vi "S_ReadAttribute.vi"(8 "error in (no error)":errorcluster, 11 "reference in":refnum<class "SubTemplate_4x4x4.lvclass">) -> (0 "error out":errorcluster, 3 "reference out":refnum<class "SubTemplate_4x4x4.lvclass">)   [LabVIEW 2012, in "SubTemplate_4x4x4.lvclass"]
uses:
  <resource>/Framework/Providers/Open_GDS/ClassProviders/Provider_EndevoGOOP300/Templates/SubTemplate_4x4x4/SubTemplate_4x4x4.lvclass
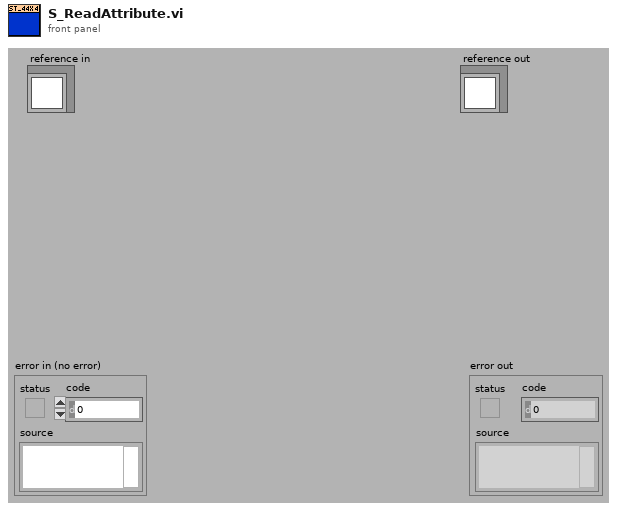
[diagram p1: front panel]
types:
  T1 = typedef "SubTemplate_4x4x4.lvclass/ObjectAttributes.ctl" = cluster{"Base class":T2}
  T2 = typedef "BaseTemplate_4x4x4.lvclass/ObjectAttributes.ctl" = cluster{"Attribute1":dbl}
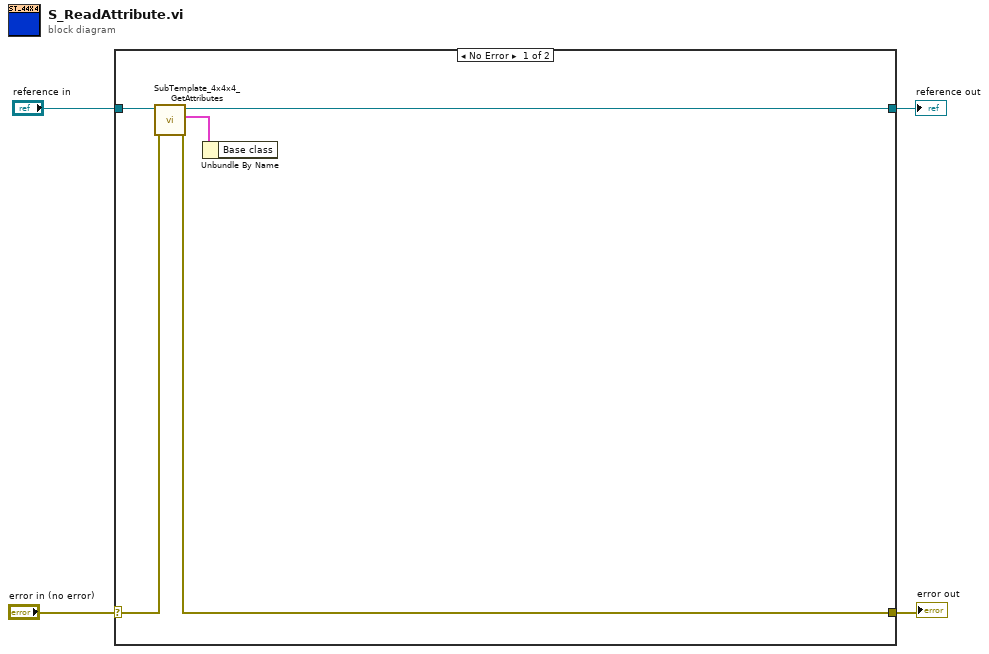
[diagram p0: block diagram]
diagram:
  n1 = case shown="No Error" "error in (no error)" {
    selector: "error in (no error)" -> [w9 w11]
    tunnel: [w7 w11] -> w3
    tunnel: [w5 w10] -> w1
    tunnel: "reference in" -> [w6 w10]
    frame No Error {
      n2 = call <resource>:"SubTemplate_4x4x4_GetAttributes.vi"("error in (no error)"=w9, "reference in"=w6) -> ("error out"=w7:errorcluster, "Attributes"=w8:T1, "reference out"=w5:refnum<class "SubTemplate_4x4x4.lvclass">)  [unwired: 6 in, 1 out]
      n3 = Unbundle By Name(w8) -> ()  [unwired: 1 out]
    }
    frame Error {
    }
  }
  "error out" <- w3
  "reference out" <- w1
